vi "ArParser.vi"(1 "from\nXMLparser":string[][](array[string]), 2 "IndicatorClasses":string[](array[string]), 3 "IndicatorTypes":string[](array[string]), 4 "IndicatorNames":string[](array[string])) -> (0 "toCreator":T1(array[cluster]))   [LabVIEW 2009]
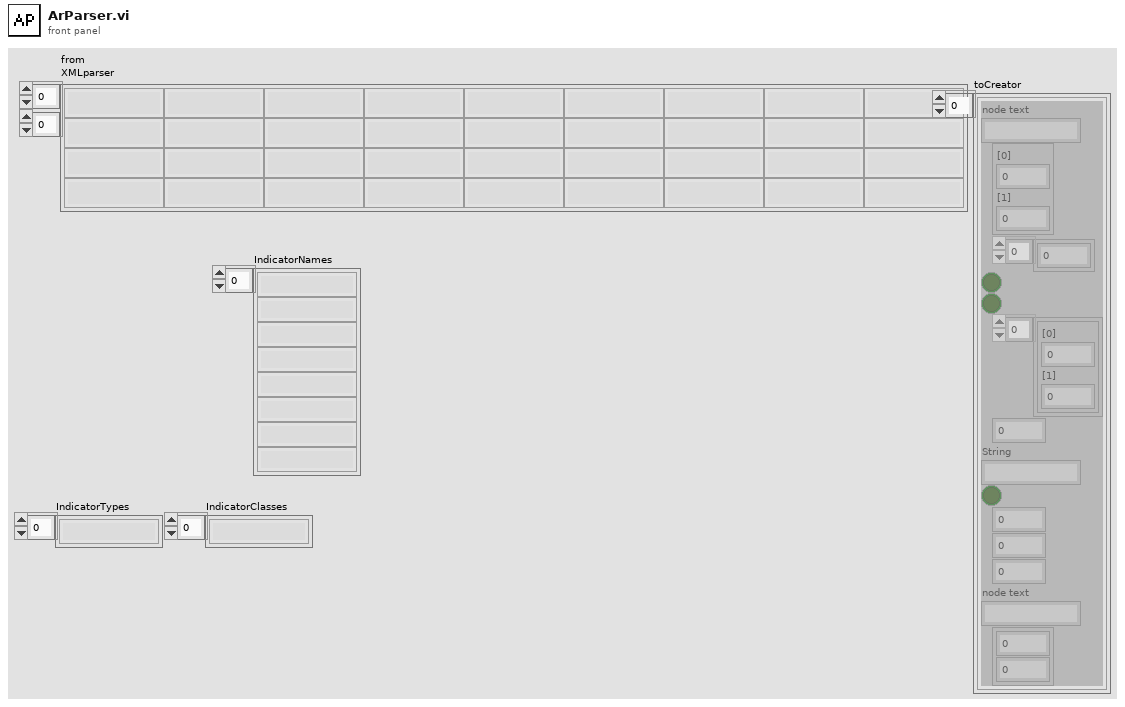
[diagram p1: front panel]
types:
  T1 = cluster{"node text":string, cluster{"[0]":i32, "[1]":i32}, i32[], bool, bool, cluster{"[0]":u32, "[1]":u32}[], i32, "String":string, bool, i32, i32, i32, "node text":string, cluster{i32, i32}}[]
  T2 = cluster{"node text":string, cluster{"[0]":i32, "[1]":i32}, "Array":i32[], "Boolean":bool, "Boolean":bool, cluster{"[0]":u32, "[1]":u32}[], i32, "String":string, bool, "Numeric":i32, "Numeric":i32, "Numeric":i32, "node text":string, cluster{"Numeric":i32, "Numeric":i32}}
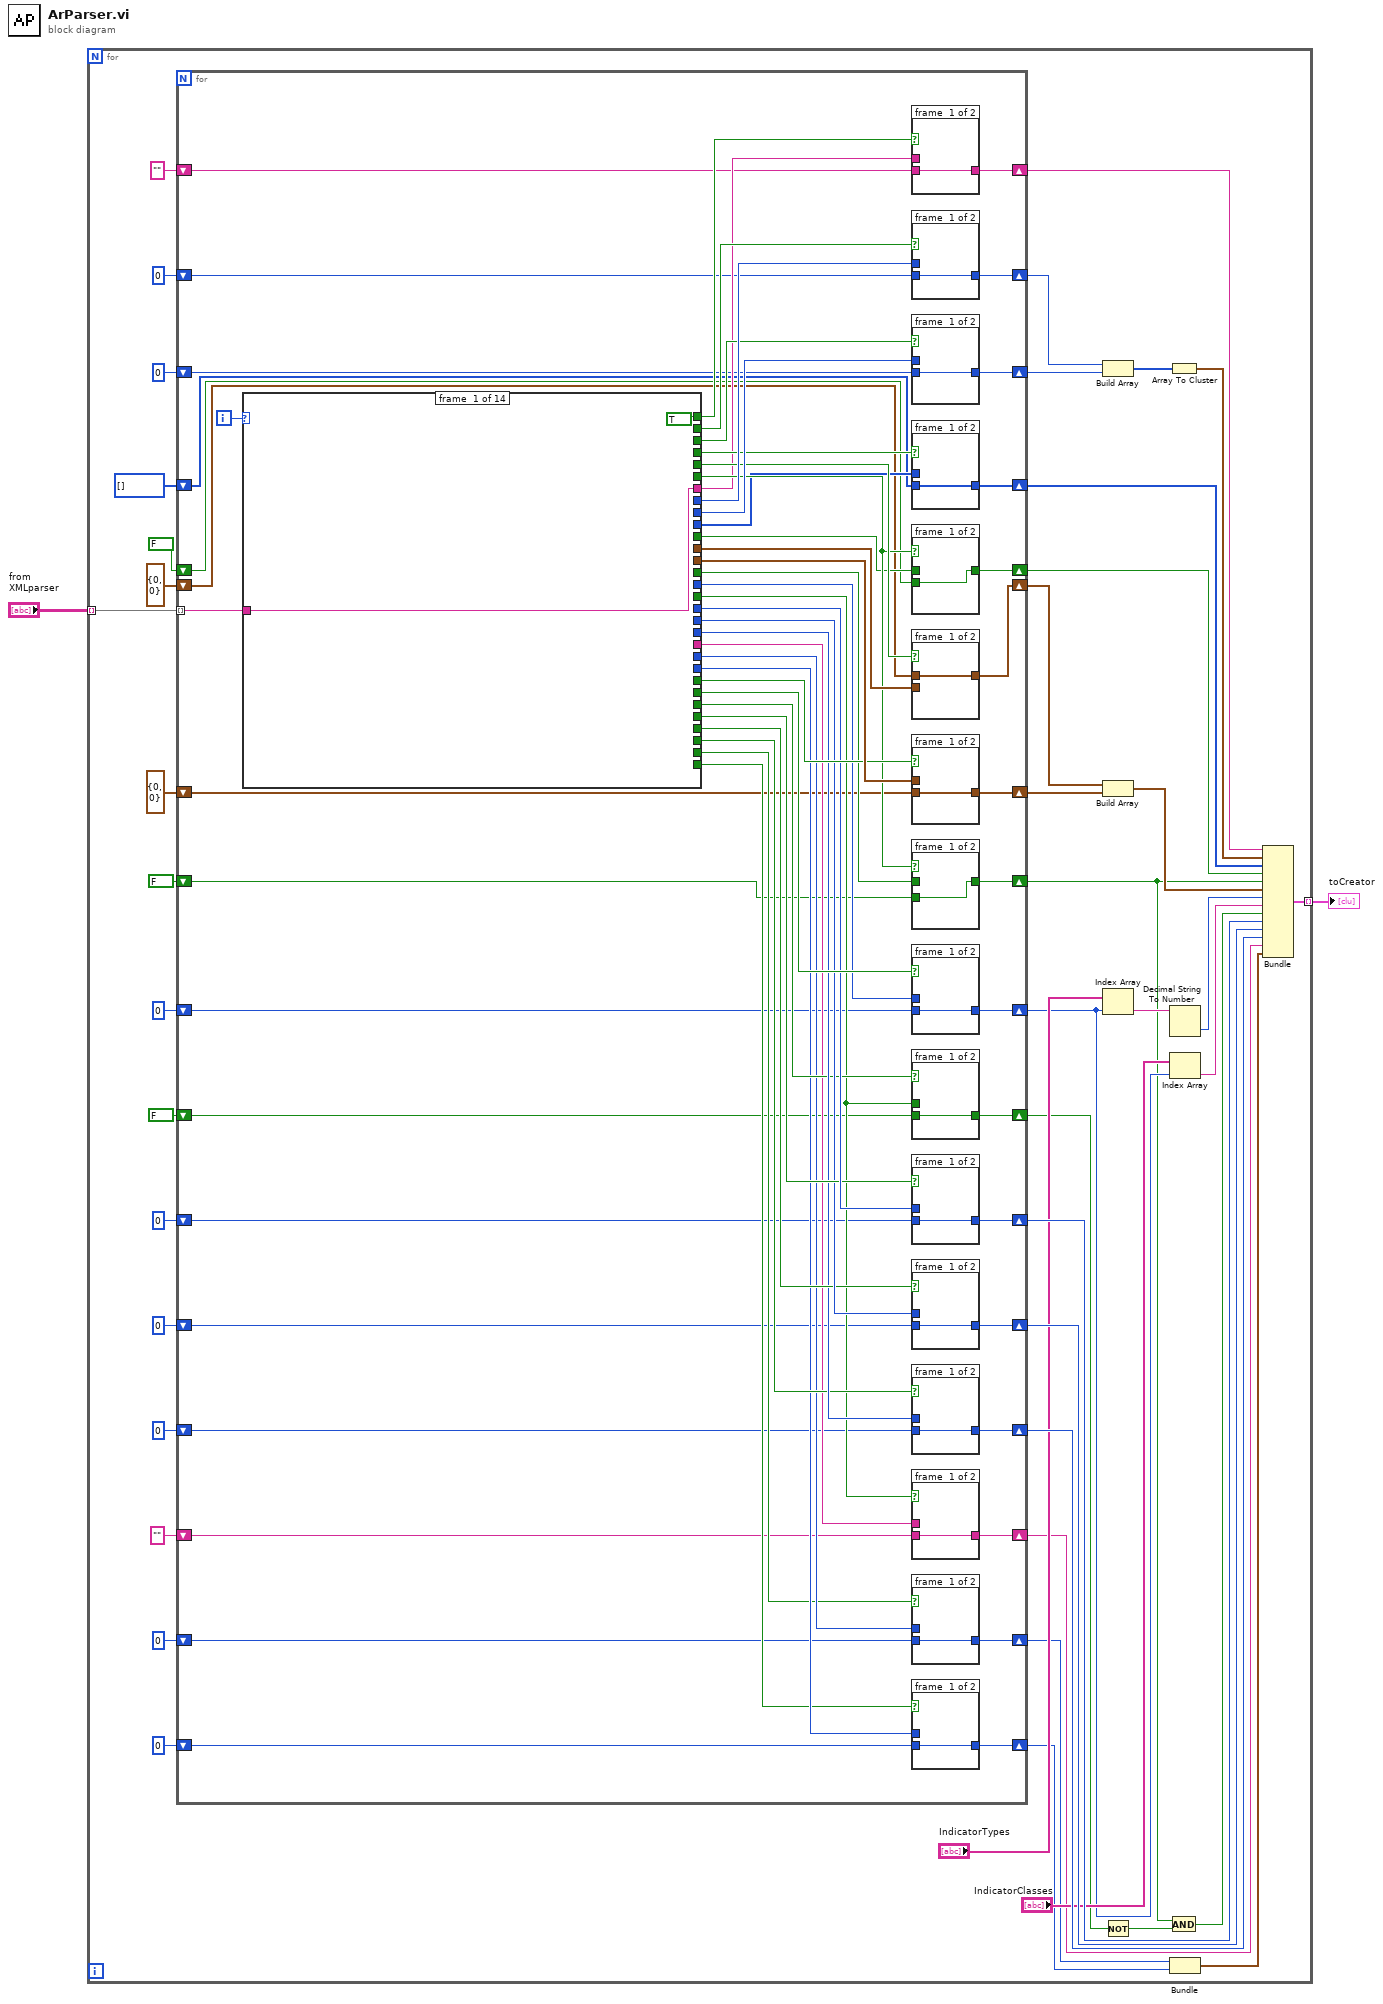
[diagram p0: block diagram]
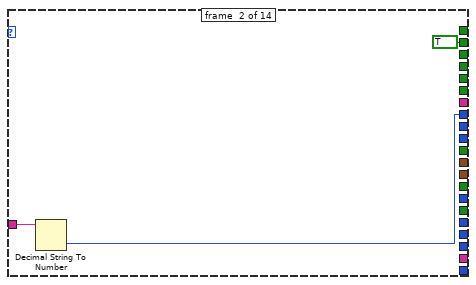
[diagram p18: hidden frame]
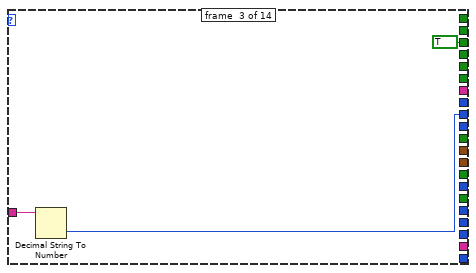
[diagram p19: hidden frame]
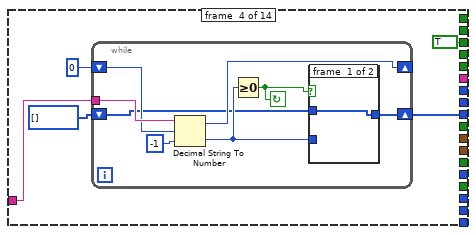
[diagram p20: hidden frame]
diagram:
  n1 = for {
    tunnel: "from\nXMLparser" -> [w47] mode=indexing
    tunnel: [w22] -> w1 mode=indexing
    n2 = for {
      tunnel: w47 -> [w111] mode=indexing
      shift-right: [w78] -> w24
      shift-left: "" ("node text") -> [w79]
      shift-right: [w76] -> w37
      shift-left: 0 ("Numeric") -> [w77]
      shift-right: [w74] -> w36
      shift-left: 0 ("Numeric") -> [w75]
      shift-right: [w72] -> w46
      shift-left: i32[] [] ("Array") -> [w73]
      shift-right: [w70] -> w45
      shift-left: FALSE ("Boolean") -> [w71]
      shift-right: [w68] -> w40
      shift-left: cluster{"[0]":u32, "[1]":u32} {"[0]"=0, "[1]"=0} ("Cluster") -> [w69]
      shift-right: [w66] -> w39
      shift-left: cluster{"[0]":u32, "[1]":u32} {"[0]"=0, "[1]"=0} ("Cluster") -> [w67]
      shift-right: [w64] -> w26
      shift-left: FALSE ("Boolean") -> [w65]
      shift-right: [w62] -> w31
      shift-left: 0 ("index of element") -> [w63]
      shift-right: [w60] -> w44
      shift-left: 0 ("Numeric") -> [w61]
      shift-right: [w58] -> w43
      shift-left: 0 ("Numeric") -> [w59]
      shift-right: [w56] -> w42
      shift-left: 0 ("Numeric") -> [w57]
      shift-right: [w54] -> w28
      shift-left: FALSE ("Boolean") -> [w55]
      shift-right: [w52] -> w23
      shift-left: "" ("node text") -> [w53]
      shift-right: [w50] -> w20
      shift-left: 0 ("Numeric") -> [w51]
      shift-right: [w48] -> w19
      shift-left: 0 ("Numeric") -> [w49]
      i -> [w106]
      n3 = case shown="3" w106 {
        tunnel: w111 -> [w144 w148 w151 w156 w170 w180 w185 w189 w195 w198 w201 w204 w207 _]
        tunnel: [w144 _ _ _ _ _ _ _ _ _ _ _ _ _] -> w92
        tunnel: [_ w147 _ _ _ _ _ _ _ _ _ _ _ _] -> w110
        tunnel: [_ _ w150 _ _ _ _ _ _ _ _ _ _ _] -> w109
        tunnel: [_ _ _ w155 _ _ _ _ _ _ _ _ _ _] -> w98
        tunnel: [_ _ _ _ w169 _ _ _ _ _ _ _ _ _] -> w99
        tunnel: [_ _ _ _ _ w177 _ _ _ _ _ _ _ _] -> w108
        tunnel: [_ _ _ _ _ _ w182 _ _ _ _ _ _ _] -> w107
        tunnel: [TRUE _ _ _ _ _ _ _ _ _ _ _ _ _] -> w105
        tunnel: [_ _ _ _ TRUE _ _ _ _ _ _ _ _ _] -> w100
        tunnel: [_ _ _ _ _ TRUE _ _ _ _ _ _ _ _] -> w104
        tunnel: [_ _ _ _ _ _ TRUE _ _ _ _ _ _ _] -> w103
        tunnel: [_ TRUE _ _ _ _ _ _ _ _ _ _ _ _] -> w102
        tunnel: [_ _ TRUE _ _ _ _ _ _ _ _ _ _ _] -> w101
        tunnel: [_ _ _ TRUE _ _ _ _ _ _ _ _ _ _] -> w97
        tunnel: [_ _ _ _ w174 _ _ _ _ _ _ _ _ _] -> w91
        tunnel: [_ _ _ _ _ _ _ w191 _ _ _ _ _ _] -> w95
        tunnel: [_ _ _ _ _ _ _ w190 _ _ _ _ _ _] -> w96
        tunnel: [_ _ _ _ _ _ _ _ w194 _ _ _ _ _] -> w94
        tunnel: [_ _ _ _ _ _ _ _ TRUE _ _ _ _ _] -> w93
        tunnel: [_ _ _ _ _ _ _ _ _ w197 _ _ _ _] -> w90
        tunnel: [_ _ _ _ _ _ _ _ _ TRUE _ _ _ _] -> w89
        tunnel: [_ _ _ _ _ _ _ _ _ _ w200 _ _ _] -> w88
        tunnel: [_ _ _ _ _ _ _ _ _ _ TRUE _ _ _] -> w87
        tunnel: [_ _ _ _ _ _ _ w186 _ _ _ _ _ _] -> w84
        tunnel: [_ _ _ _ _ _ _ w190 _ _ _ _ _ _] -> w86
        tunnel: [_ _ _ _ _ _ _ w189 _ _ _ _ _ _] -> w85
        tunnel: [_ _ _ _ _ _ _ _ _ _ _ w203 _ _] -> w83
        tunnel: [_ _ _ _ _ _ _ _ _ _ _ TRUE _ _] -> w82
        tunnel: [_ _ _ _ _ _ _ _ _ _ _ _ w206 _] -> w81
        tunnel: [_ _ _ _ _ _ _ _ _ _ _ _ TRUE _] -> w80
        frame #0 {
        }
        frame #1 {
          n4 = Decimal String To Number(string=w148) -> (number=w147:i32)  [unwired: 2 in, 1 out]
        }
        frame #2 {
          n5 = Decimal String To Number(string=w151) -> (number=w150:i32)  [unwired: 2 in, 1 out]
        }
        frame #3 {
          n6 = while {
            tunnel: w156 -> [w164]
            shift-right: [w163] -> _
            shift-left: 0 ("offset past number") -> [w162]
            shift-right: [w157] -> w155
            shift-left: i32[] [] ("Array") -> [w158]
            stop <- w160 continue-if-true
            n7 = Decimal String To Number(string=w164, offset=w162, default (0L)=-1 ("default (0 I32)")) -> (offset past number=w163:i32, number=w159:i32)
            n8 = Greater Or Equal To 0?(x=w159) -> (x >= 0?=w160:bool)
            n9 = case shown="True" w160 {
              tunnel: w158 -> [w165 w167]
              tunnel: w159 -> [_ w166]
              tunnel: [w165 w168] -> w157
              frame #0 {
              }
              frame #1 {
                n10 = Build Array (concatenate)(w167, w166) -> (w168:i32[])
              }
            }
          }
        }
        frame #4 {
          n11 = Equal?(x=w170, y="in") -> (x = y?=w169:bool)
          n12 = Equal?(x="out", y=w170) -> (x = y?=w171:bool)
          n13 = Or(x=w171, y=w169) -> (x .or. y?=w174:bool)
        }
        frame #5 {
          n14 = Hexadecimal String To Number(string=w180) -> (number=w176:u32)  [unwired: 2 in, 1 out]
          n15 = Build Array(w176, w176) -> (w178:u32[])
          n16 = Array To Cluster(array=w178) -> (cluster=w177:cluster{"[0]":u32, "[1]":u32})
        }
        frame #6 {
          n17 = Hexadecimal String To Number(string=w185) -> (number=w181:u32)  [unwired: 2 in, 1 out]
          n18 = Build Array(w181, w181) -> (w183:u32[])
          n19 = Array To Cluster(array=w183) -> (cluster=w182:cluster{"[0]":u32, "[1]":u32})
        }
        frame #7 {
          w190 = TRUE
          n20 = Search 1D Array(1D array="IndicatorNames", element=w189) -> (index of element=w188:i32)  [unwired: 1 in]
          n21 = Increment(x=w188) -> (x+1=w187:i32)
          n22 = Less Than 0?(x=w188) -> (x < 0?=w186:bool)
          n23 = Select(t=w187, s=w186, f=w188) -> (s? t:f=w191:i32)
        }
        frame #8 {
          n24 = Decimal String To Number(string=w195) -> (number=w194:i32)  [unwired: 2 in, 1 out]
        }
        frame #9 {
          n25 = Decimal String To Number(string=w198) -> (number=w197:i32)  [unwired: 2 in, 1 out]
        }
        frame #10 {
          n26 = Decimal String To Number(string=w201) -> (number=w200:i32)  [unwired: 2 in, 1 out]
        }
        frame #11 {
          n27 = Decimal String To Number(string=w204) -> (number=w203:i32)  [unwired: 2 in, 1 out]
        }
        frame #12 {
          n28 = Decimal String To Number(string=w207) -> (number=w206:i32)  [unwired: 2 in, 1 out]
        }
        frame #13 {
        }
      }
      n29 = case shown="True" w105 {
        tunnel: w79 -> [w142 _]
        tunnel: w92 -> [_ w143]
        tunnel: [w142 w143] -> w78
        frame #0 {
        }
        frame #1 {
        }
      }
      n30 = case shown="True" w102 {
        tunnel: w77 -> [w140 _]
        tunnel: w110 -> [_ w141]
        tunnel: [w140 w141] -> w76
        frame #0 {
        }
        frame #1 {
        }
      }
      n31 = case shown="True" w101 {
        tunnel: w75 -> [w138 _]
        tunnel: w109 -> [_ w139]
        tunnel: [w138 w139] -> w74
        frame #0 {
        }
        frame #1 {
        }
      }
      n32 = case shown="True" w97 {
        tunnel: w73 -> [w136 _]
        tunnel: w98 -> [_ w137]
        tunnel: [w136 w137] -> w72
        frame #0 {
        }
        frame #1 {
        }
      }
      n33 = case shown="True" w100 {
        tunnel: w71 -> [w134 _]
        tunnel: w99 -> [_ w135]
        tunnel: [w134 w135] -> w70
        frame #0 {
        }
        frame #1 {
        }
      }
      n34 = case shown="True" w103 {
        tunnel: w67 -> [w130 _]
        tunnel: w107 -> [_ w131]
        tunnel: [w130 w131] -> w66
        frame #0 {
        }
        frame #1 {
        }
      }
      n35 = case shown="True" w104 {
        tunnel: w69 -> [w132 _]
        tunnel: w108 -> [_ w133]
        tunnel: [w132 w133] -> w68
        frame #0 {
        }
        frame #1 {
        }
      }
      n36 = case shown="True" w100 {
        tunnel: w65 -> [w128 _]
        tunnel: w91 -> [_ w129]
        tunnel: [w128 w129] -> w64
        frame #0 {
        }
        frame #1 {
        }
      }
      n37 = case shown="True" w96 {
        tunnel: w63 -> [w126 _]
        tunnel: w95 -> [_ w127]
        tunnel: [w126 w127] -> w62
        frame #0 {
        }
        frame #1 {
        }
      }
      n38 = case shown="True" w86 {
        tunnel: w55 -> [w118 _]
        tunnel: w84 -> [_ w119]
        tunnel: [w118 w119] -> w54
        frame #0 {
        }
        frame #1 {
        }
      }
      n39 = case shown="True" w93 {
        tunnel: w61 -> [w124 _]
        tunnel: w94 -> [_ w125]
        tunnel: [w124 w125] -> w60
        frame #0 {
        }
        frame #1 {
        }
      }
      n40 = case shown="True" w89 {
        tunnel: w59 -> [w122 _]
        tunnel: w90 -> [_ w123]
        tunnel: [w122 w123] -> w58
        frame #0 {
        }
        frame #1 {
        }
      }
      n41 = case shown="True" w87 {
        tunnel: w57 -> [w120 _]
        tunnel: w88 -> [_ w121]
        tunnel: [w120 w121] -> w56
        frame #0 {
        }
        frame #1 {
        }
      }
      n42 = case shown="True" w84 {
        tunnel: w53 -> [w116 _]
        tunnel: w85 -> [_ w117]
        tunnel: [w116 w117] -> w52
        frame #0 {
        }
        frame #1 {
        }
      }
      n43 = case shown="True" w80 {
        tunnel: w49 -> [w112 _]
        tunnel: w81 -> [_ w113]
        tunnel: [w112 w113] -> w48
        frame #0 {
        }
        frame #1 {
        }
      }
      n44 = case shown="True" w82 {
        tunnel: w51 -> [w114 _]
        tunnel: w83 -> [_ w115]
        tunnel: [w114 w115] -> w50
        frame #0 {
        }
        frame #1 {
        }
      }
    }
    n45 = Build Array(w37, w36) -> (w38:i32[])
    n46 = Build Array(w39, w40) -> (w41:cluster{"[0]":u32, "[1]":u32}[])
    n47 = Index Array(array="IndicatorTypes", index=w31) -> (element=w32:string)
    n48 = Not(x=w28) -> (.not. x?=w27:bool)
    n49 = Array To Cluster(array=w38) -> (cluster=w35:cluster{"[0]":i32, "[1]":i32})
    n50 = And(x=w26, y=w27) -> (x .and. y?=w25:bool)
    n51 = Decimal String To Number(string=w32) -> (number=w30:i32)  [unwired: 2 in, 1 out]
    n52 = Index Array(array="IndicatorClasses", index=w31) -> (element=w29:string)
    n53 = Bundle("Numeric"=w19, "Numeric"=w20) -> (w21:cluster{"Numeric":i32, "Numeric":i32})  [unwired: 1 in]
    n54 = Bundle("node text"=w24, w35, "Array"=w46, "Boolean"=w45, "Boolean"=w26, w41, w30, "String"=w29, w25, "Numeric"=w44, "Numeric"=w43, "Numeric"=w42, "node text"=w23, w21) -> (w22:T2)  [unwired: 1 in]
  }
  "toCreator" <- w1
